vi "Lakeshore 336 Test Program.vi"() -> ()   [LabVIEW 2024, in "Lakeshore 336.lvclass"]
uses:
  Lakeshore 336.lvclass
  Lakeshore 336 Channel Settings cluster.ctl
  Lakeshore 336 PID cluster.ctl
  <instrlib>/Lake Shore 336/Lake Shore 336.lvlib
panel:
  in  "Manual Settings":T1={"Input (0:None)"=1, "Power Up Enable (F: Off)"=FALSE, "Mode (0:Off)"=1, "Max Current (0:User Specified)"=0, "Heater Out Display (1:Current)"=1, "Max User Current (2.000)"=2.0, "Heater Resistance (1:25 Ohms)"=2, "PID"={"P"=0.1, "I"=0.0, "D"=0.0}, "Name"="Test"} {"Heater Resistance (1:25 Ohms)" items=["25 Ohms"=1, "50 Ohms"=2]; "Max User Current (2.000)" format="%.3f"; "Heater Out Display (1:Current)" items=["Current"=1, "Power"=2]; "Max Current (0:User Specified)" items=["User Specified", "0.707 A", "1.0 A", "1.141 A", "2.0 A"]; "Mode (0:Off)" items=["Off", "Closed Loop PID", "Zone", "Open Loop"]; "Input (0:None)" items=["None", "A", "B", "C", "D"]}
  in  "Output (1:1)":u16(ring)=1 items=["1"=1, "2"=2, "3"=3, "4"=4]
  out "error out":errorcluster
  in  "VISA resource name":refnum<visa-resource-name>="TCPIP0::192.168.121.12::7777::SOCKET"
  out "Setpoint":dbl format="%.5f"
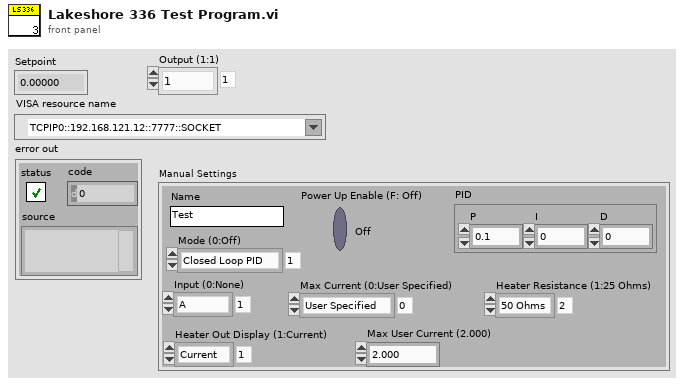
[diagram p1: front panel]
types:
  T1 = typedef "Lakeshore 336.lvclass/Lakeshore 336 Channel Settings cluster.ctl" = cluster{"Input (0:None)":u16, "Power Up Enable (F: Off)":bool, "Mode (0:Off)":u16, "Max Current (0:User Specified)":u16, "Heater Out Display (1:Current)":u16, "Max User Current (2.000)":dbl, "Heater Resistance (1:25 Ohms)":u16, "PID":T2, "Name":string}
  T2 = typedef "Lakeshore 336.lvclass/Lakeshore 336 PID cluster.ctl" = cluster{"P":dbl, "I":dbl, "D":dbl}
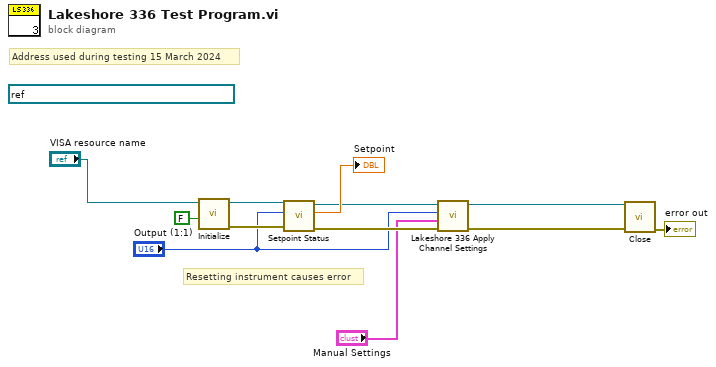
[diagram p0: block diagram]
diagram:
  (unwired) refnum<visa-resource-name> "TCPIP0::192.168.121.12::7777::SOCKET" ("VISA resource name")
  # "Address used during testing 15 March 2024"
  # "Resetting instrument causes error"
  n1 = call <instrlib>:"Initialize.vi"("Reset (True)"=FALSE, "VISA resource name"="VISA resource name") -> ("error out"=w9:errorcluster, "VISA resource name out"=w12:refnum<visa-resource-name>)  [unwired: 8 in]
  n2 = call <instrlib>:"Setpoint Status.vi"("error in (no error)"=w9, "Output (1:1)"="Output (1:1)", "VISA resource name"=w12) -> ("error out"=w5:errorcluster, "Setpoint"=→"Setpoint":dbl, "VISA resource name out"=w6:refnum<visa-resource-name>)  [unwired: 6 in]
  n3 = call "Lakeshore 336 Apply Channel Settings.vi"("error in (no error)"=w5, "Manual Settings"="Manual Settings", "Channel (1)"="Output (1:1)", "Addr"=w6) -> ("error out"=w3:errorcluster, "Addr dup"=w4:refnum<visa-resource-name>)  [unwired: 5 in, 1 out]
  n4 = call <instrlib>:"Close.vi"("error in (no error)"=w3, "VISA resource name"=w4) -> ("error out"=→"error out":errorcluster)  [unwired: 9 in]
